vi "resistancePIP.vi"(8 "error in (no error)":errorcluster, 9 "DeviceType":string, 10 "QUICK_KEYS":bool, 11 "RESISTANCE":bool) -> (0 "error out":errorcluster, 3 "RESISTANCE-15":string)   [LabVIEW 2018]
uses:
  Global_1259.vi
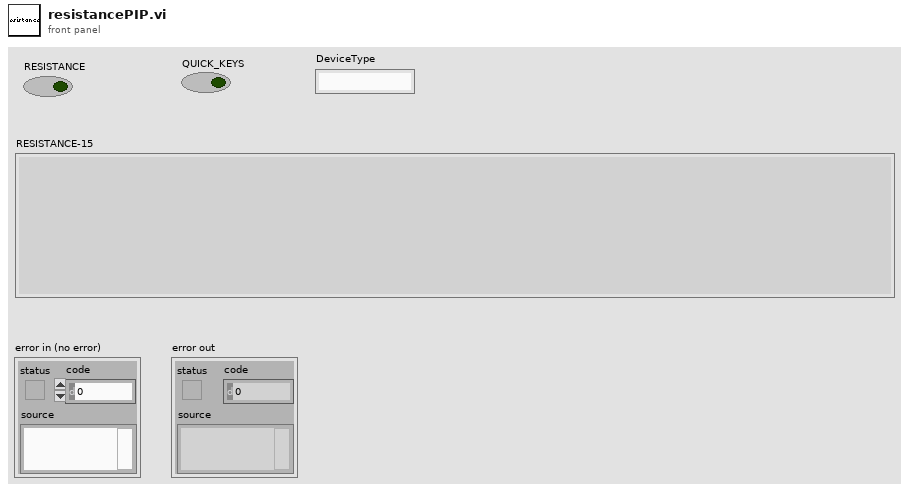
[diagram p1: front panel]
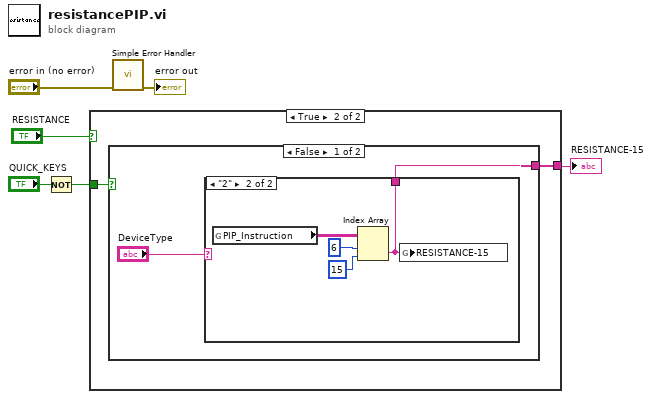
[diagram p0: block diagram]
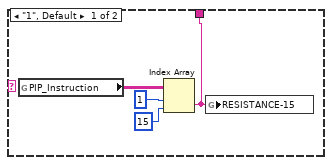
[diagram p3: hidden frame]
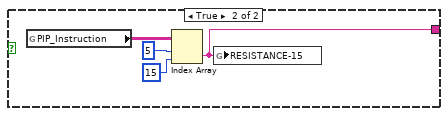
[diagram p4: hidden frame]
diagram:
  n1 = Not(x="QUICK_KEYS") -> (.not. x?=w1:bool)
  n2 = case shown="True" "RESISTANCE" {
    tunnel: w1 -> [_ w8]
    tunnel: [_ w7] -> w2
    frame False {
    }
    frame True {
      n3 = case shown="False" w8 {
        tunnel: [w10 w19] -> w7
        frame False {
          n4 = case shown="\"2\"" "DeviceType" {
            tunnel: [w11 w15] -> w10
            frame "1", Default {
              n5 = global read "Global_1259.vi" "PIP_Instruction"() -> (w14:string[][])
              n6 = Index Array(array=w14, index (row)=1, index (col)=15 ("disabled index (col)")) -> (element=w11:string)
              n7 = global write "Global_1259.vi" "RESISTANCE-15"(w11) -> ()
            }
            frame "2" {
              n8 = global read "Global_1259.vi" "PIP_Instruction"() -> (w18:string[][])
              n9 = Index Array(array=w18, index (row)=6, index (col)=15 ("disabled index (col)")) -> (element=w15:string)
              n10 = global write "Global_1259.vi" "RESISTANCE-15"(w15) -> ()
            }
          }
        }
        frame True {
          n11 = global read "Global_1259.vi" "PIP_Instruction"() -> (w22:string[][])
          n12 = Index Array(array=w22, index (row)=5, index (col)=15 ("disabled index (col)")) -> (element=w19:string)
          n13 = global write "Global_1259.vi" "RESISTANCE-15"(w19) -> ()
        }
      }
    }
  }
  "RESISTANCE-15" <- w2
  n14 = call <vilib>:"Simple Error Handler.vi"("error in (no error)"="error in (no error)") -> ("error out"=→"error out":errorcluster)  [unwired: 4 in, 4 out]
